vi "RT Main.vi"() -> ()   [LabVIEW 2018]
panel:
  out "data out":dbl[][](array[numeric])
  out "timed out?":bool
  out "available IP addresses":string[](array[string])
  out "number of addresses":i32
  # "RT reader"
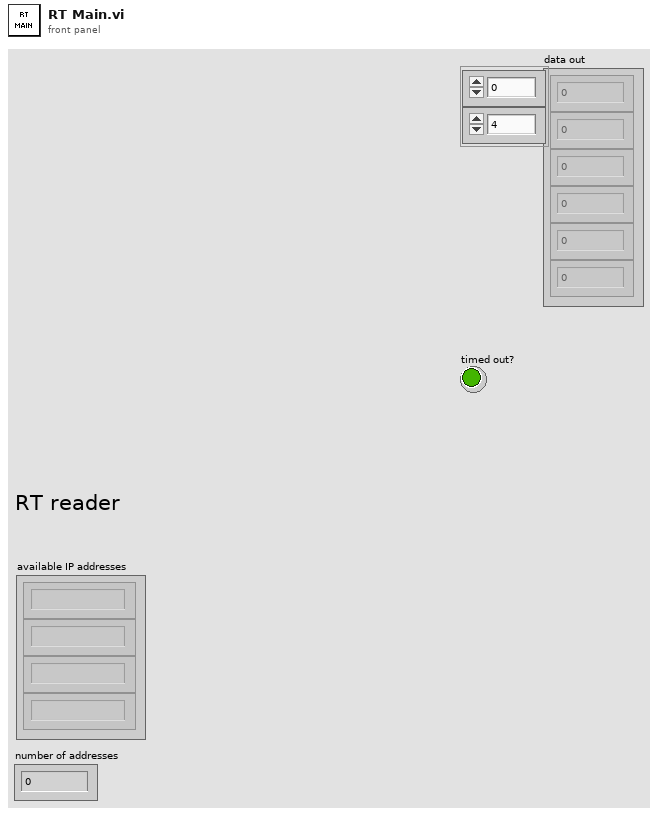
[diagram p1: front panel]
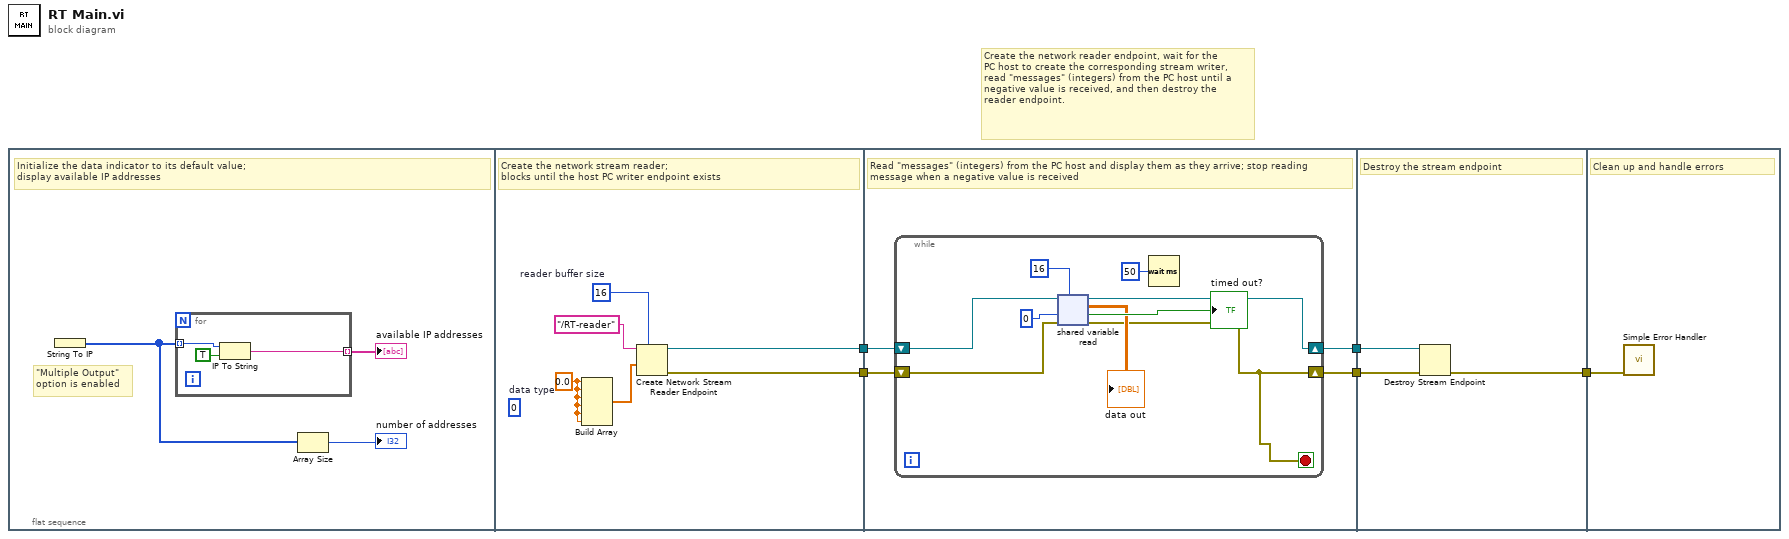
[diagram p0: block diagram]
diagram:
  # "Create the network reader endpoint, wait for the\nPC host to create the corresponding stream writer,\nread \"messages\" (integers) from the PC host until a\nnegative value is received, and then destroy the \nreader endpoint."
  n1 = flat-sequence {
    tunnel: [w15] -> w3
    tunnel: [w14] -> w2
    tunnel: [w18] -> w5
    tunnel: [w19] -> w4
    tunnel: w3 -> [w20]
    tunnel: w2 -> [w21]
    tunnel: w5 -> [w33]
    tunnel: w4 -> [w32]
    tunnel: [w31] -> w1
    tunnel: w1 -> [w34]
    frame #0 {
      # "\"Multiple Output\"\noption is enabled"
      # "Initialize the data indicator to its default value;\ndisplay available IP addresses"
      n2 = String To IP() -> (0:w6:u32[])  [unwired: 1 in]
      n3 = for {
        tunnel: w6 -> [w10] mode=indexing
        tunnel: [w9] -> w7 mode=indexing
        n4 = IP To String(1:TRUE ("dot notation? (F)"), 2:w10) -> (0:w9:string)
      }
      "available IP addresses" <- w7
      n5 = Array Size(array=w6) -> (size(s)=→"number of addresses":i32)
    }
    frame #1 {
      w12 = 0.0 ("element")
      (unwired) 0  # data type
      w17 = 16  # reader buffer size
      # "Create the network stream reader;\nblocks until the host PC writer endpoint exists"
      n6 = Build Array(w12, w12, w12, w12, w12, w12) -> (w13:dbl[])
      n7 = Create Network Stream Reader Endpoint(7:w17, 9:w13, 11:"/RT-reader" ("writer name")) -> (0:w15:errorcluster, 3:w14:refnum<k21>)  [unwired: 4 in]
    }
    frame #2 {
      # "Read \"messages\" (integers) from the PC host and display them as they arrive; stop reading message when a negative value is received"
      n8 = while {
        shift-right: [w28] -> w18
        shift-left: w21 -> [w30]
        shift-right: [w22] -> w19
        shift-left: w20 -> [w27]
        stop <- w22 stop-if-true
        n9 = shared-variable-read(w30, w27, 0 ("timeout ms (-1)"), 16 ("# elements")) -> (w28:refnum<k21>, w22:errorcluster, →"timed out?":bool, →"data out":dbl[][])
        n10 = Wait (ms)(milliseconds to wait=u32 50) -> ()  [unwired: 1 out]
      }
    }
    frame #3 {
      # "Destroy the stream endpoint"
      n11 = Destroy Stream Endpoint(8:w32, 11:w33) -> (0:w31:errorcluster)
    }
    frame #4 {
      # "Clean up and handle errors"
      n12 = call <vilib>:"Simple Error Handler.vi"("error in (no error)"=w34) -> ()  [unwired: 4 in, 5 out]
    }
  }
